vi "Operation Main.vi"(8 "error in (no error)":errorcluster, 11 "Display Actor in":refnum<class "Display Actor.lvclass">) -> (0 "error out":errorcluster, 3 "Display Actor out":refnum<class "Display Actor.lvclass">)   [LabVIEW 2024, in "Display Actor.lvclass"]
uses:
  Display Actor.lvclass
  Ancestor Class/Actor/System Actor/System Actor.lvclass
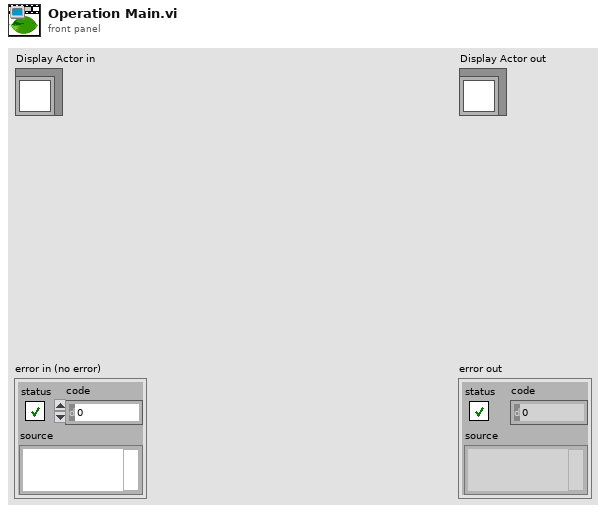
[diagram p1: front panel]
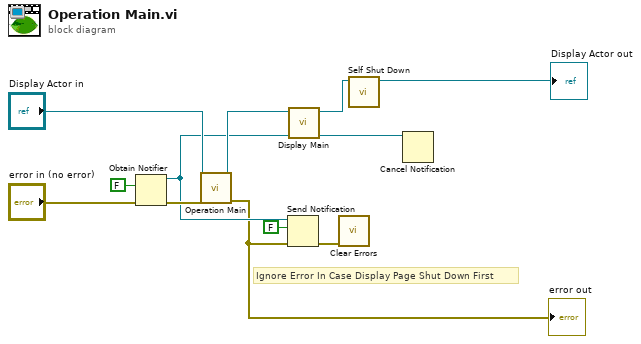
[diagram p0: block diagram]
diagram:
  # "Ignore Error In Case Display Page Shut Down First"
  n1 = Obtain Notifier(notification data type=FALSE, error in (no error)="error in (no error)") -> (notifier out=w6:refnum<notifier>, error out=w10:errorcluster)  [unwired: 2 in, 1 out]
  n2 = call-parent "Operation Main.vi"("error in (no error)"=w10, "System Actor in"="Display Actor in") -> ("error out"=w2:errorcluster, "System Actor out"=w7:refnum<class "Display Actor.lvclass">)  [unwired: 8 in]
  "error out" <- w2
  n3 = Send Notification(notification=FALSE, notifier=w6, error in (no error)=w2) -> (error out=w1:errorcluster)  [unwired: 1 out]
  n4 = call-dynamic "Display Main.vi"("Stop Notifier In"=w6, "Display Actor in"=w7) -> ("Stop Notifier Out"=w5:refnum<notifier>, "Display Actor out"=w4:refnum<class "Display Actor.lvclass">)  [unwired: 8 in]
  n5 = call <vilib>:"Clear Errors.vi"("error in (no error)"=w1) -> ()  [unwired: 5 in, 2 out]
  n6 = call-dynamic "Self Shut Down.vi"("Display Actor in"=w4) -> ("Display Actor out"=→"Display Actor out":refnum<class "Display Actor.lvclass">)  [unwired: 10 in]
  n7 = Cancel Notification(0:w5) -> ()  [unwired: 1 in, 3 out]
